vi "ConvertCalculateFormatElementsToItemList.vi"(11 "Calculate Format Elements":T1[](array[typedef])) -> (3 "Item List":string)   [LabVIEW 8.6, in "Keithley-6482-Visa.lvlib"]
uses:
  Keithley-6482-Visa.lvlib
  Public/Controls/CalculateFormatElement.ctl
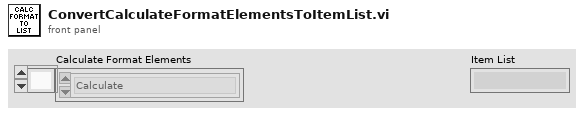
[diagram p1: front panel]
types:
  T1 = typedef "Keithley-6482-Visa.lvlib/CalculateFormatElement.ctl" = enum16{"Calculate", "Time", "Status"}
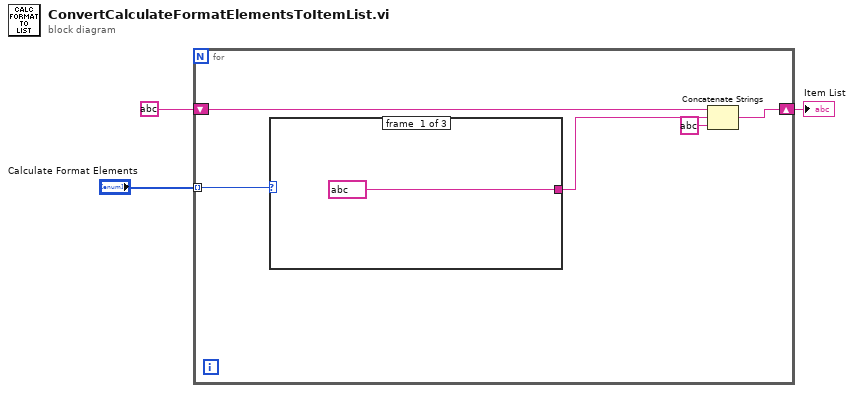
[diagram p0: block diagram]
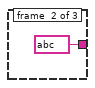
[diagram p2: hidden frame]
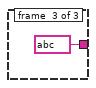
[diagram p3: hidden frame]
diagram:
  n1 = for {
    tunnel: "Calculate Format Elements" -> [w6] mode=indexing
    shift-right: [w7] -> w1
    shift-left: string ? -> [w8]
    n2 = case shown="\"Status\"" w6 {
      tunnel: [string ? string ? string ?] -> w5
      frame #0 {
      }
      frame #1 {
      }
      frame #2 {
      }
    }
    n3 = Concatenate Strings(w8, w5, string ? ("string")) -> (w7:string)
  }
  "Item List" <- w1
